vi "INICIA_SERIAL_AQUISICAO_QUEUED.vi"() -> ()   [LabVIEW 2018]
uses:
  Global_Telescopio.vi
  <vilib>/Instr/_visa.llb/VISA Configure Serial Port (Instr).vi
panel:
  out "AQUISICAO  RESOURCE":refnum<visa-resource-name>
  in  "flow control (0:none)":u16(ring) items=["None", "XON/XOFF", "RTS/CTS", "XON/XOFF & RTS/CTS", "DTR/DSR", "XON/XOFF & DTR/DSR"]
  in  "stop bits (10: 1 bit)":u16(ring)=10 items=["1.0"=10, "1.5"=15, "2.0"=20]
  in  "parity (0:none)":enum16{"None", "Odd", "Even", "Mark", "Space"}(ring)
  in  "baud rate (2400)":u32=2400
  in  "VISA resource name":refnum<visa-resource-name>="COM65"
  # "COM 65 NECESSÁRIA"
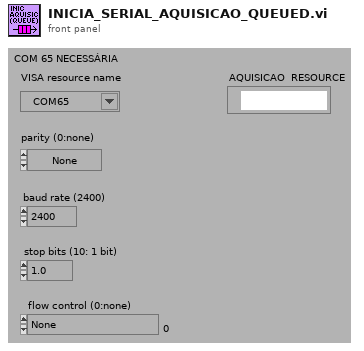
[diagram p1: front panel]
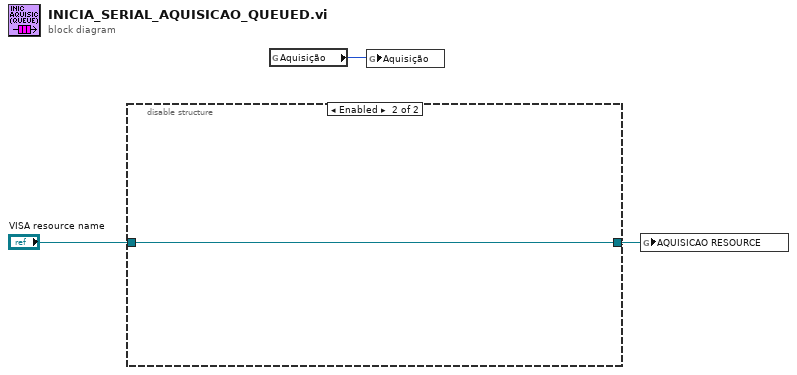
[diagram p0: block diagram]
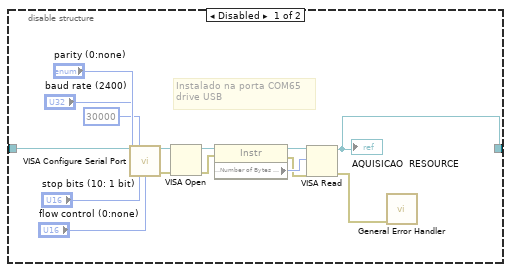
[diagram p2: hidden frame]
diagram:
  n1 = disable-structure shown="Enabled" {
    disable-tunnel: "VISA resource name" -> [w6 w19]
    disable-tunnel: [w4 w19] -> w2
    frame Disabled {
      # "Instalado na porta COM65\ndrive USB"
      n2 = call-poly "VISA Configure Serial Port"("VISA resource name"=w6, "timeout (10sec)"=u32 30000, "baud rate (9600)"="baud rate (2400)", "parity (0:none)"="parity (0:none)", "stop bits (10: 1 bit)"="stop bits (10: 1 bit)", "flow control (0:none)"="flow control (0:none)") -> ("VISA resource name out"=w12:refnum<visa-resource-name>, "error out"=w13:errorcluster)  [unwired: 8 in]
      n3 = VISA Open(error in (no error)=w13, VISA resource name=w12) -> (VISA resource name=w17:refnum<visa-resource-name>, error out=w18:errorcluster)  [unwired: 3 in]
      n4 = property class="Instr"(reference=w17, error in=w18) -> (reference out=w14:refnum<visa-resource-name>, error out=w15:errorcluster, "Serial Settings:Number of Bytes at Serial Port"=w16:u32)
      n5 = VISA Read(VISA resource name=w14, byte count=w16, error in (no error)=w15) -> (VISA resource name out=w4:refnum<visa-resource-name>, error out=w5:errorcluster)  [unwired: 2 out]
      "AQUISICAO  RESOURCE" <- w4
      n6 = call <vilib>:"General Error Handler.vi"("error in (no error)"=w5) -> ()  [unwired: 10 in, 5 out]
    }
    frame Enabled {
    }
  }
  n7 = global read "Global_Telescopio.vi" "Aquisição"() -> (w1:i32)
  n8 = global write "Global_Telescopio.vi" "Aquisição"(w1) -> ()
  n9 = global write "Global_Telescopio.vi" "AQUISICAO RESOURCE"(w2) -> ()
